vi "setRoot.vi"(8 "error in (no error)":errorcluster, 10 "Root":refnum<data-value>, 11 "Tree in":refnum<class "Tree.lvclass">) -> (0 "error out":errorcluster, 3 "Tree out":refnum<class "Tree.lvclass">)   [LabVIEW 2009, in "Tree.lvclass"]
doc: "Set the root of the tree."
uses:
  Tree.lvclass
  TreeNode/TreeNode.lvclass
  Tree.lvclass/Tree.ctl
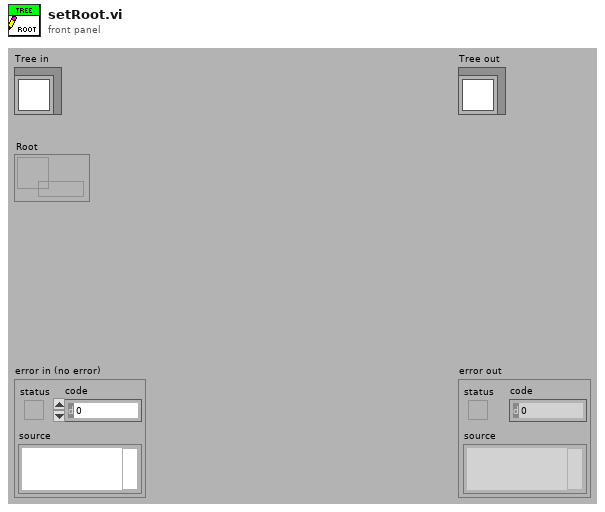
[diagram p1: front panel]
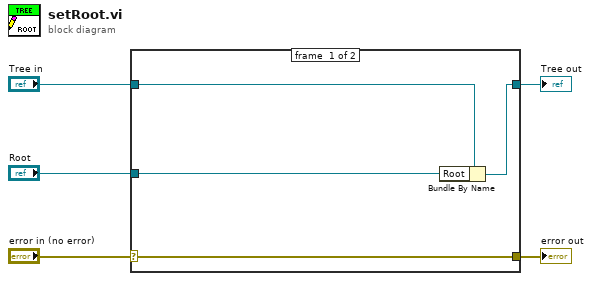
[diagram p0: block diagram]
diagram:
  n1 = case shown="No Error" "error in (no error)" {
    selector: "error in (no error)" -> [w9 w10]
    tunnel: [w9 w10] -> w4
    tunnel: [w7 w11] -> w2
    tunnel: "Tree in" -> [w8 w11]
    tunnel: "Root" -> [w6 _]
    frame #0 {
      n2 = Bundle By Name(cluster=w8, "Root"=w6) -> (w7:refnum<class "Tree.lvclass">)
    }
    frame #1 {
    }
  }
  "error out" <- w4
  "Tree out" <- w2
